vi "Write Outgoing Frame.vi"(7 "opcode":T1=2 items=["continuation"=0, "text"=1, "binary"=2, "close"=8, "ping"=9, "pong"=10], 8 "error in (no error)":errorcluster, 9 "timeout ms (2000)":i32=2000, 10 "Bytes":u8[](array[numeric]) format="%08b", 11 "Connection.WS":refnum<class "Connection.WS.lvclass">) -> (0 "error out":errorcluster, 3 "Connection.WS":refnum<class "Connection.WS.lvclass">)   [LabVIEW 2013, in "Connection.WS_GOSPL.lvlib" / "Connection.WS.lvclass"]
uses:
  Connection.WS.lvclass
  Websocket Frame Type -- ring.ctl
  Connection/Connection.lvclass/Connection.ctl
  Connection/Connection.lvclass
  Connection.TCP/Connection.TCP.lvclass
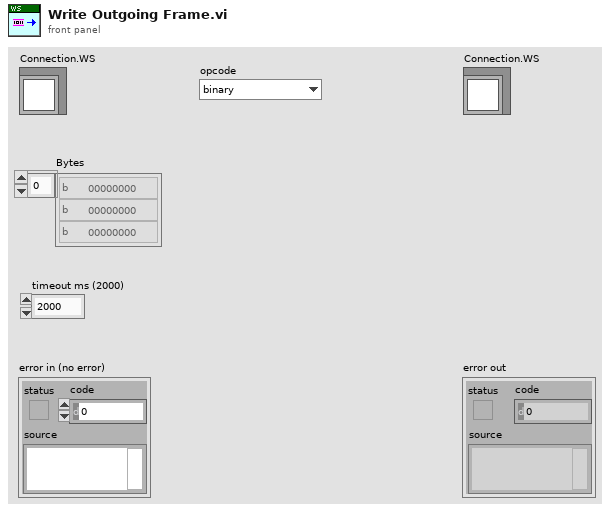
[diagram p1: front panel]
types:
  T1 = typedef "Connection.WS_GOSPL.lvlib/Connection.WS.lvclass/Websocket Frame Type -- ring.ctl" = u8
  T2 = cluster{"state":enum16{"generate mask", "compute payload length", "send payload", "end"}, "final-fragment":bool, "opcode":T1, "masked":bool, "mask":u8[], "length":u8[]}
  T3 = enum16{"generate mask", "compute payload length", "send payload", "end"}
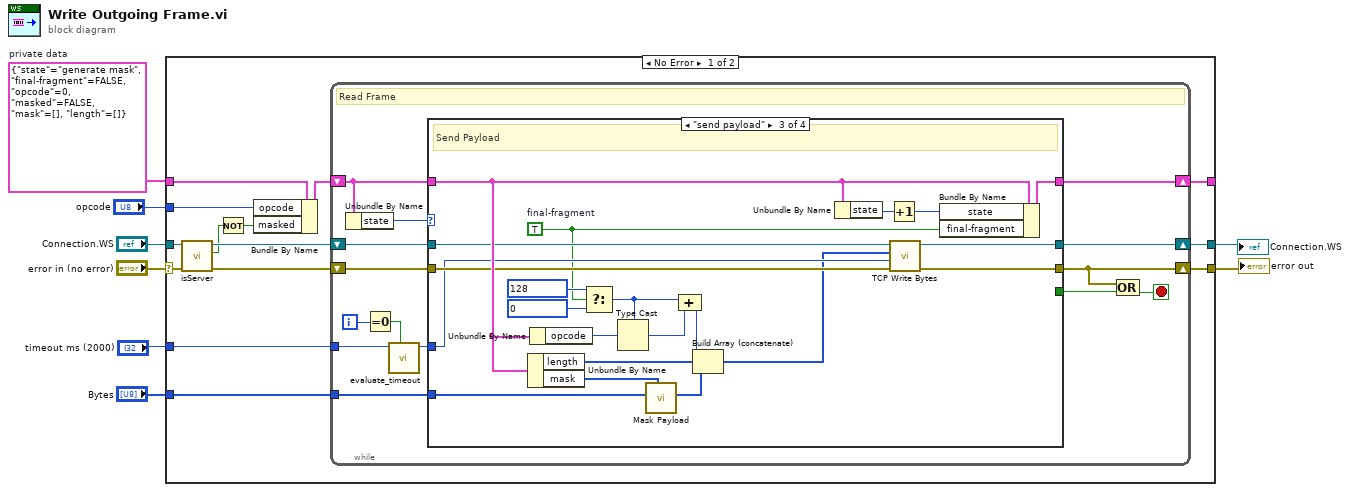
[diagram p0: block diagram]
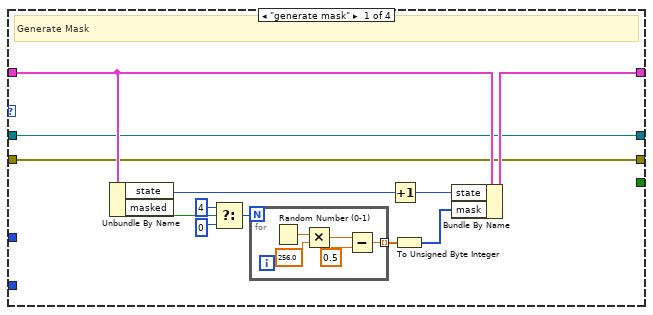
[diagram p2: hidden frame]
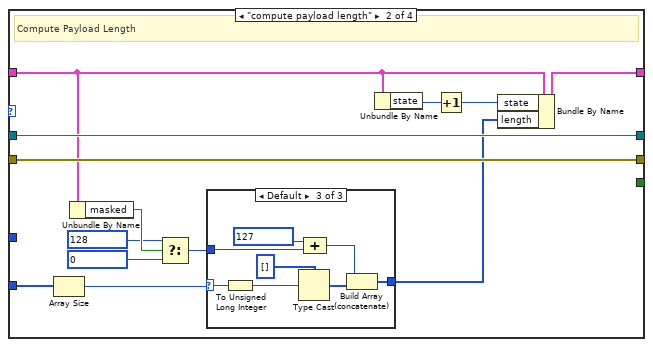
[diagram p3: hidden frame]
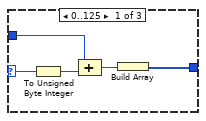
[diagram p4: hidden frame]
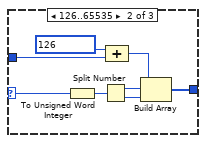
[diagram p5: hidden frame]
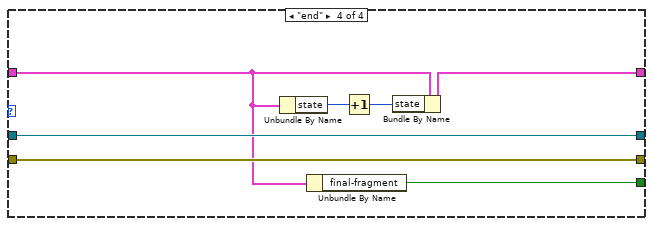
[diagram p6: hidden frame]
diagram:
  w8 = T2 {"state"=enum."generate mask", "final-fragment"=FALSE, "opcode"=0, "masked"=FALSE, "mask"=[], "length"=[]}  # private data
  n1 = case shown="No Error" "error in (no error)" {
    selector: "error in (no error)" -> [w18 w116]
    tunnel: "Connection.WS" -> [w16 w117]
    tunnel: [w22 w117] -> w3
    tunnel: [w21 w116] -> w4
    tunnel: "timeout ms (2000)" -> [w20 _]
    tunnel: w8 -> [w14 _]
    tunnel: [w19 _] -> _
    tunnel: "opcode" -> [w12 _]
    tunnel: "Bytes" -> [w9 _]
    frame No Error {
      n2 = call "isServer.vi"("error in (no error)"=w18, "Connection in"=w16) -> ("error out"=w17:errorcluster, "server"=w11:bool, "Connection out"=w15:refnum<class "Connection.WS.lvclass">)  [unwired: 7 in]
      n3 = Not(x=w11) -> (.not. x?=w10:bool)
      n4 = Bundle By Name(cluster=w14, "opcode"=w12, "masked"=w10) -> (w13:T2)
      n5 = while {
        shift-right: [w30] -> w22
        shift-left: w15 -> [w34]
        shift-right: [w31] -> w21
        shift-left: w17 -> [w32]
        tunnel: w20 -> [w35]
        shift-right: [w26] -> w19
        shift-left: w13 -> [w25]
        tunnel: w9 -> [w23]
        i -> [w27]
        stop <- w36 stop-if-true
        # "Read Frame"
        n6 = Unbundle By Name(w25) -> ("state"=w24:T3)
        n7 = Equal To 0?(x=w27) -> (x = 0?=w29:bool)
        n8 = call "evaluate_timeout.vi"("reset?"=w29, "timeout (ms)"=w35) -> ("remaining timeout (ms)"=w33:i32)  [unwired: 8 in, 1 out]
        n9 = case shown="\"send payload\"" w24 {
          tunnel: w34 -> [w44 w63 w103 w115]
          tunnel: w33 -> [_ _ w99 _]
          tunnel: w32 -> [w43 w62 w100 w114]
          tunnel: [w43 w62 w101 w114] -> w31
          tunnel: [w44 w63 w102 w115] -> w30
          tunnel: [_ _ _ w112] -> w28
          tunnel: w25 -> [w47 w61 w104 w109]
          tunnel: [w48 w66 w106 w113] -> w26
          tunnel: w23 -> [_ w60 w98 _]
          frame "generate mask" {
            # "Generate Mask"
            n10 = Unbundle By Name(w47) -> ("state"=w46:T3, "masked"=w40:bool)
            n11 = Select(t=4, s=w40, f=0) -> (s? t:f=w38:i32)
            n12 = for {
              N: w38 -> [_]
              tunnel: [w50] -> w42 mode=indexing
              n13 = Random Number (0-1)() -> (number: 0 to 1=w53:dbl)
              n14 = Multiply(x=w53, y=256.0) -> (x*y=w51:dbl)
              n15 = Subtract(x=w51, y=0.5) -> (x-y=w50:dbl)
            }
            n16 = Increment(x=w46) -> (x+1=w45:T3)
            n17 = To Unsigned Byte Integer(number=w42) -> (unsigned 8bit integer=w41:u8[])
            n18 = Bundle By Name(cluster=w47, "state"=w45, "mask"=w41) -> (w48:T2)
          }
          frame "compute payload length" {
            # "Compute Payload Length"
            n19 = Array Size(array=w60) -> (size(s)=w59:i32)
            n20 = Unbundle By Name(w61) -> ("masked"=w58:bool)
            n21 = Select(t=u8 128, s=w58, f=u8 0) -> (s? t:f=w55:u8)
            n22 = case shown="Default" w59 {
              selector: w59 -> [w71 w72 w83]
              tunnel: w55 -> [w70 w77 w85]
              tunnel: [w67 w78 w86] -> w54
              frame 0..125 {
                n23 = To Unsigned Byte Integer(number=w71) -> (unsigned 8bit integer=w69:u8)
                n24 = Compound Arithmetic op=ADD(w70, w69) -> (w68:u8)
                n25 = Build Array(w68) -> (w67:u8[])
              }
              frame 126..65535 {
                n26 = To Unsigned Word Integer(number=w72) -> (unsigned 16bit integer=w75:u16)
                n27 = Split Number(x=w75) -> (hi(x)=w74:u8, lo(x)=w73:u8)
                n28 = Compound Arithmetic op=ADD(u8 126, w77) -> (w79:u8)
                n29 = Build Array(w79, w74, w73) -> (w78:u8[])
              }
              frame Default {
                n30 = To Unsigned Long Integer(number=w83) -> (unsigned 32bit integer=w82:u32)
                n31 = Type Cast(type=u8[] [] ("payload"), x=w82) -> (*(type *) &x=w80:u8[])
                n32 = Compound Arithmetic op=ADD(u8 127, w85) -> (w87:u8)
                n33 = Build Array (concatenate)(w87, w80) -> (w86:u8[])
              }
            }
            n34 = Unbundle By Name(w61) -> ("state"=w65:T3)
            n35 = Increment(x=w65) -> (x+1=w64:T3)
            n36 = Bundle By Name(cluster=w61, "state"=w64, "length"=w54) -> (w66:T2)
          }
          frame "send payload" {
            w93 = TRUE  # final-fragment
            # "Send Payload"
            n37 = Unbundle By Name(w104) -> ("length"=w91:u8[], "mask"=w105:u8[])
            n38 = Unbundle By Name(w104) -> ("opcode"=w90:T1)
            n39 = Select(t=u8 128, s=w93, f=u8 0) -> (s? t:f=w89:u8)
            n40 = Type Cast(type=w89, x=w90) -> (*(type *) &x=w88:u8)
            n41 = call "Mask Payload.vi"("mask"=w105, "Input"=w98) -> ("Output"=w97:u8[])  [unwired: 9 in]
            n42 = Compound Arithmetic op=ADD(w89, w88) -> (w92:u8)
            n43 = Build Array (concatenate)(w92, w91, w97) -> (w96:u8[])
            n44 = Unbundle By Name(w104) -> ("state"=w108:T3)
            n45 = Increment(x=w108) -> (x+1=w107:T3)
            n46 = call "TCP Write Bytes.vi"("error in (no error)"=w100, "timeout ms (2000)"=w99, "Bytes"=w96, "Connection.TCP"=w103) -> ("error out"=w101:errorcluster, "Connection.TCP"=w102:refnum<class "Connection.WS.lvclass">)  [unwired: 6 in]
            n47 = Bundle By Name(cluster=w104, "state"=w107, "final-fragment"=w93) -> (w106:T2)
          }
          frame "end" {
            n48 = Unbundle By Name(w109) -> ("state"=w111:T3)
            n49 = Unbundle By Name(w109) -> ("final-fragment"=w112:bool)
            n50 = Increment(x=w111) -> (x+1=w110:T3)
            n51 = Bundle By Name(cluster=w109, "state"=w110) -> (w113:T2)
          }
        }
        n52 = Compound Arithmetic op=OR(w31, w28) -> (w36:bool)
      }
    }
    frame Error {
    }
  }
  "error out" <- w4
  "Connection.WS" <- w3
